vi "hts_commands.vi"(8 "Error IN":errorcluster, 9 "EXP SETTINGS":refnum<notifier>, 10 "SETTINGS":refnum<notifier>, 11 "COMMAND":T1) -> (0 "error out":errorcluster, 1 "EXP Settings":refnum<notifier>, 2 "Settings":refnum<notifier>)   [LabVIEW 2013]
uses:
  main_machine/type_defs/global_settings.ctl
  main_machine/type_defs/experiment_settings.ctl
  main_machine/type_defs/experiment_states.ctl
  type_defs/hts_command_list.ctl
panel:
  out "current command":T1
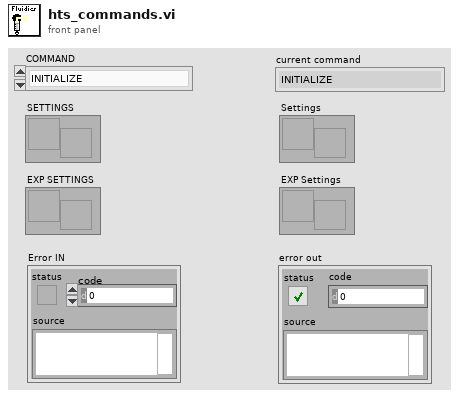
[diagram p1: front panel]
types:
  T1 = typedef "hts_command_list.ctl" = enum16{"INITIALIZE", "ADD MEDIA", "ADD INDUCER", "REMOVE CULTURE", "SAMPLE REACTOR", "CLEAR LINE TO VALVE", "CLEAR LINE TO CYTOMETER", "SAMPLE REACTOR NO DILUTION"}
  T2 = typedef "global_settings.ctl" = cluster{"# REACTORS":u32, "17X PORT":i32, "WASTE POSITION ":i32, "SECONDS BETWEEN SAMPLING":dbl, "FACS DIVA DIRECTORY":path, "DATA FILE":path, "REACTORS TO USE":u32[], "PULSE PERIOD":i32, "USE LIGHTS?":bool, "LED FILE":path, "LED CHANNELS":u32[], "PULSE LENGTH":i32, "SUMMARY FILE":path, "OUTGROWTH TIME POINTS":dbl, "SELECTION VALVE PORT":refnum<visa-resource-name>, "HTS PORT":refnum<visa-resource-name>, "DILUTION VOLUME (uL)":i32, "DILUTION FILE":path, "1X PORT":i32}
  T3 = typedef "experiment_settings.ctl" = cluster{"fcs file byte offset":i64, "LED Device Handle Out":u32, "START TIME":timestamp, "CURRENT VALVE":u32, "SAMPLE #":i32, "FCS FILE PATH":path, "TIME POINT":i32, "STATE":T4, "TIME TILL SAMPLE":dbl, "DILUTION  TABLE":dbl[][]}
  T4 = typedef "experiment_states.ctl" = enum16{"OUTGROWTH", "INDUCTION", "EXPERIMENT"}
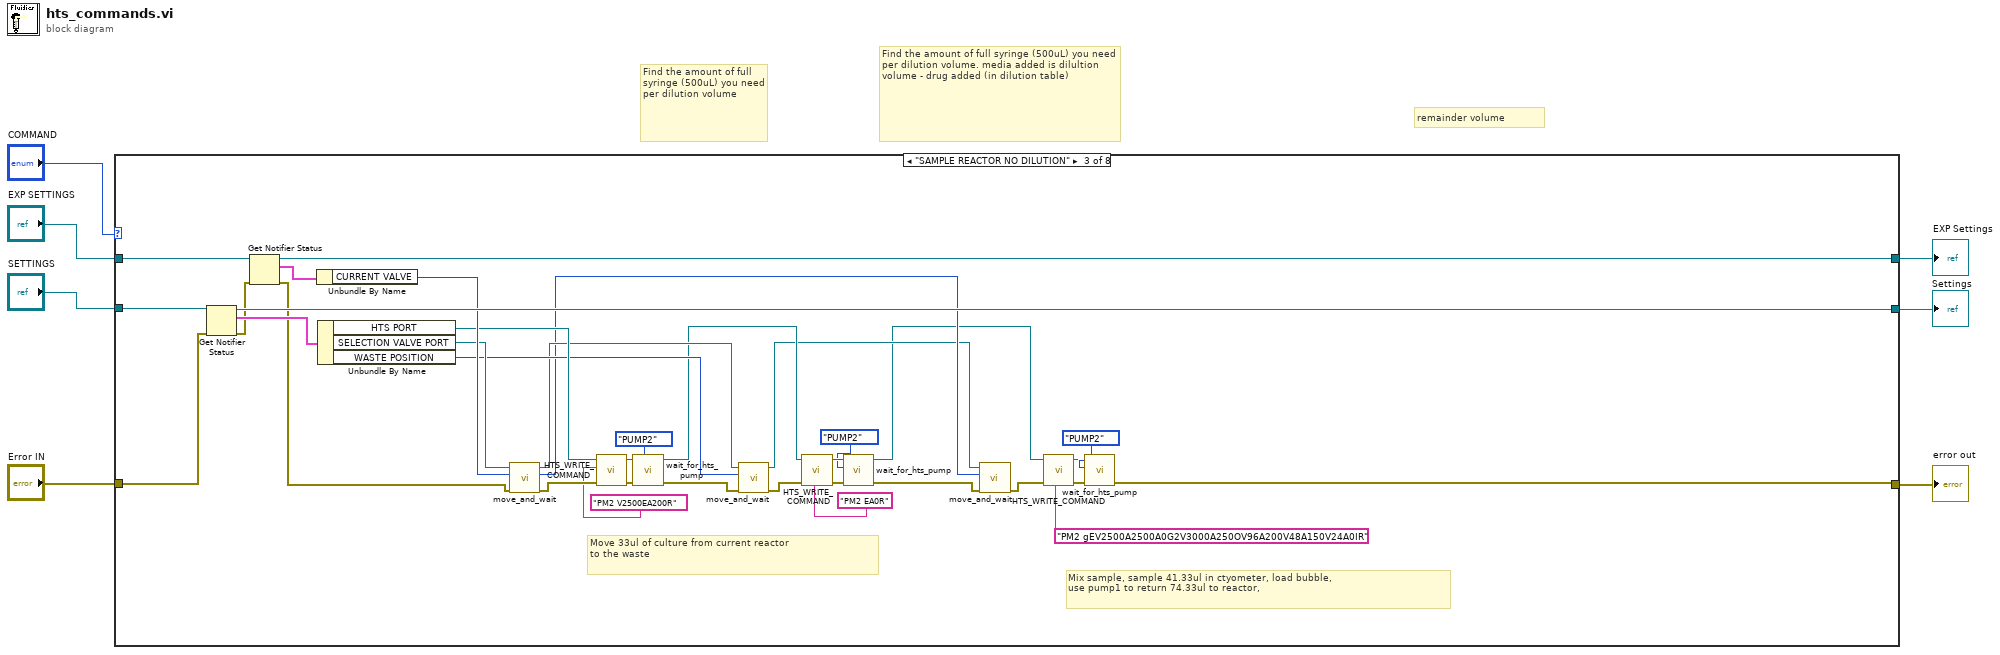
[diagram p0: block diagram]
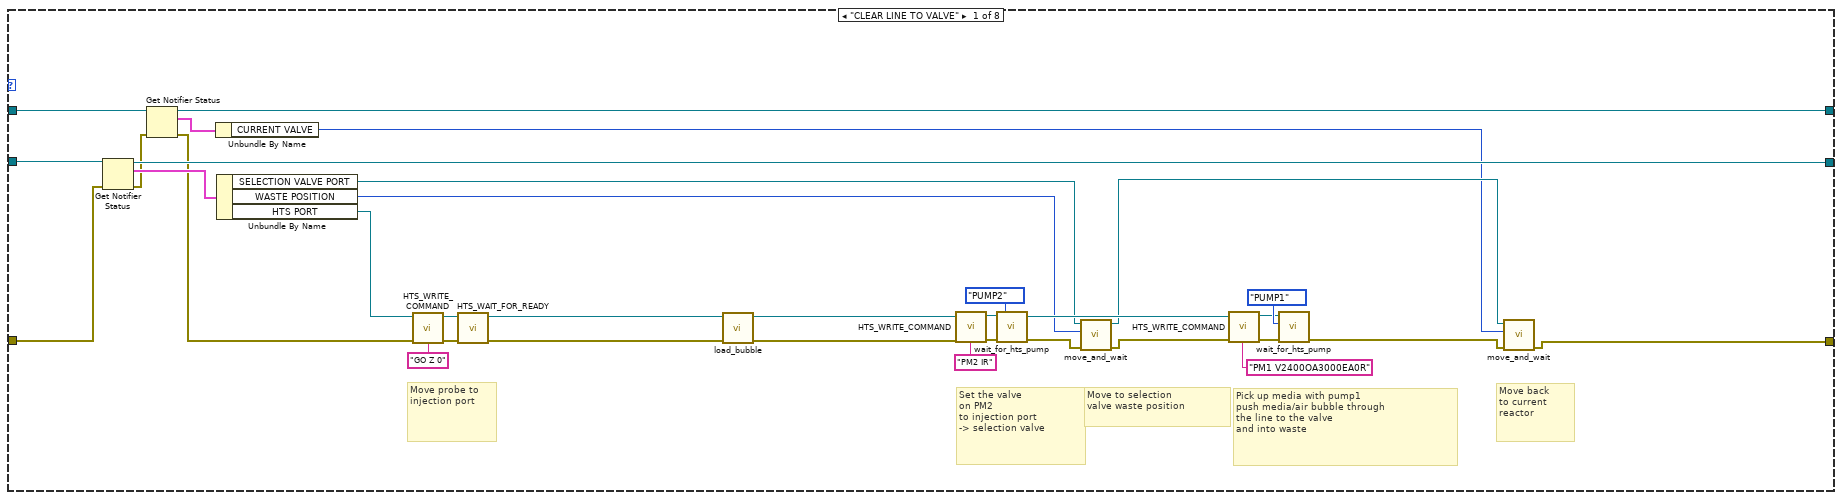
[diagram p2: hidden frame]
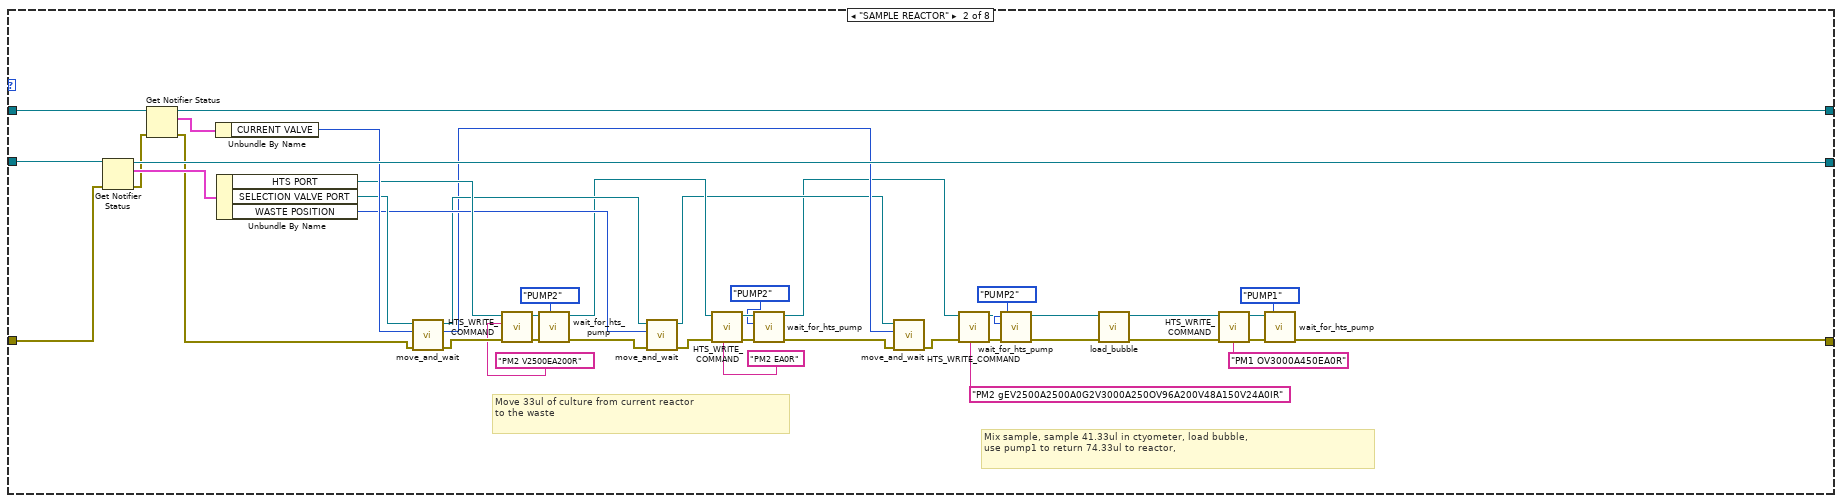
[diagram p3: hidden frame]
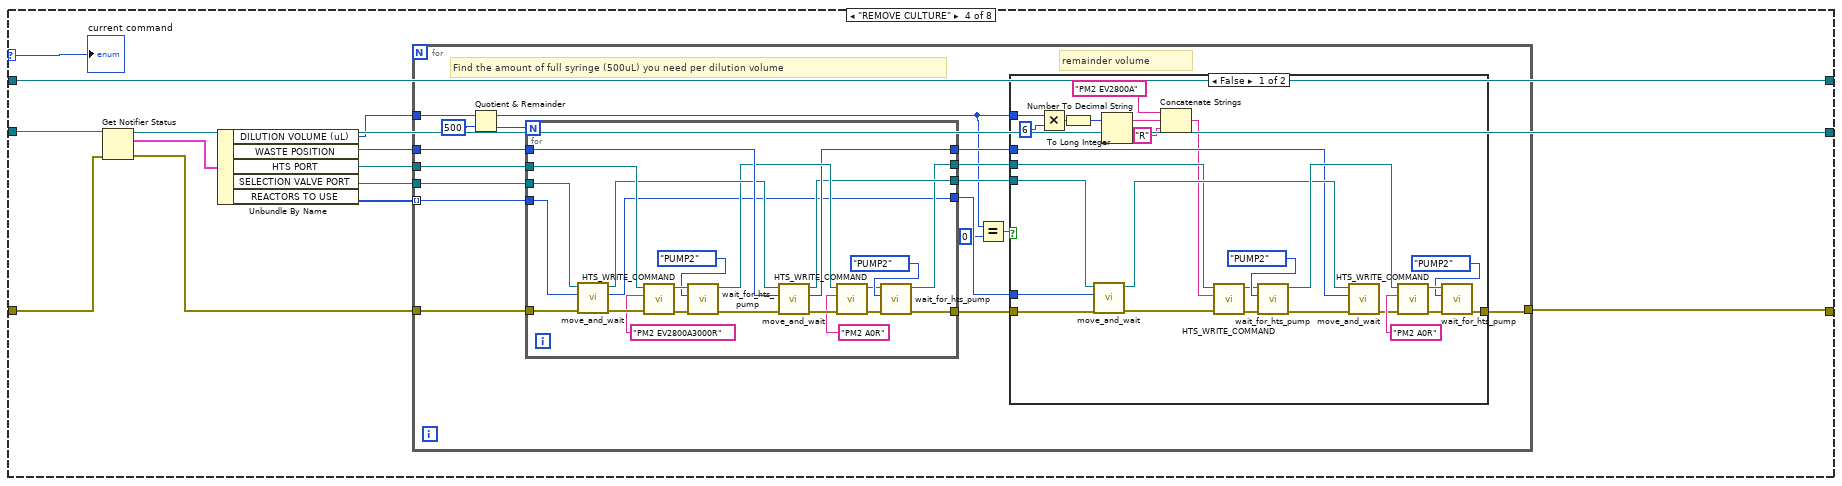
[diagram p4: hidden frame]
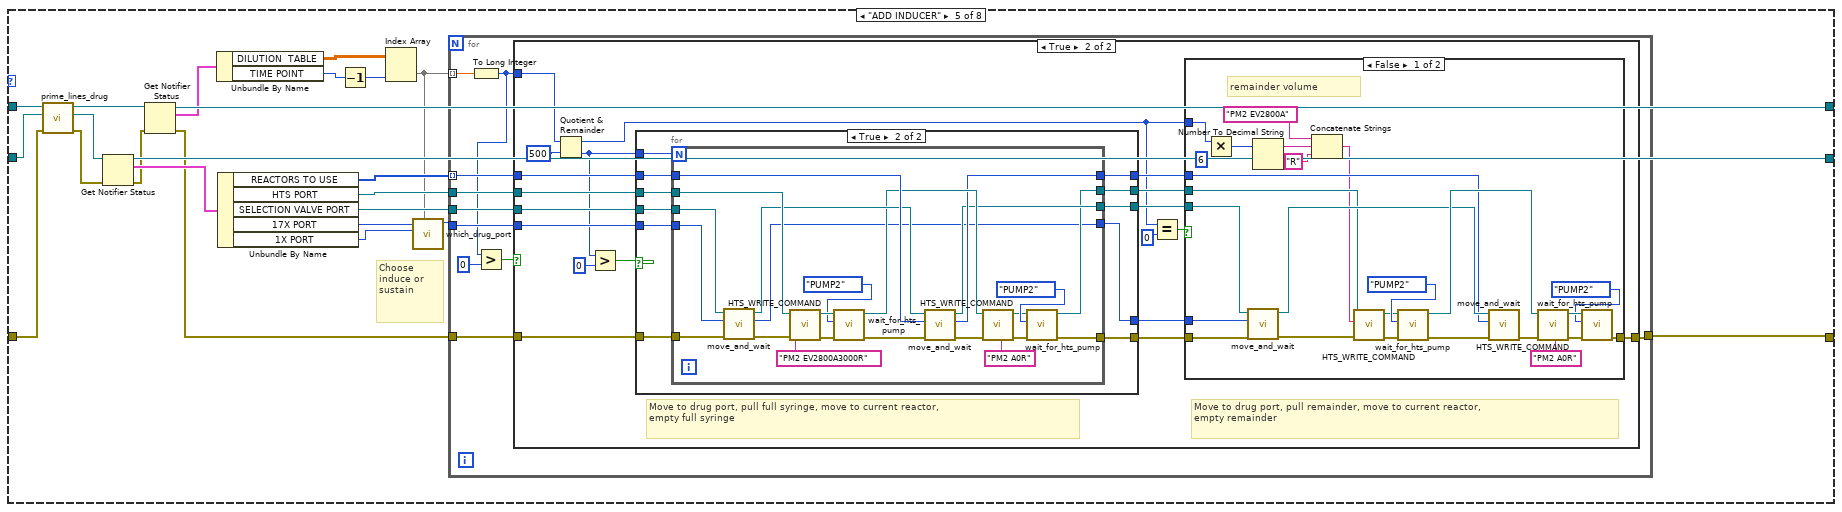
[diagram p6: hidden frame]
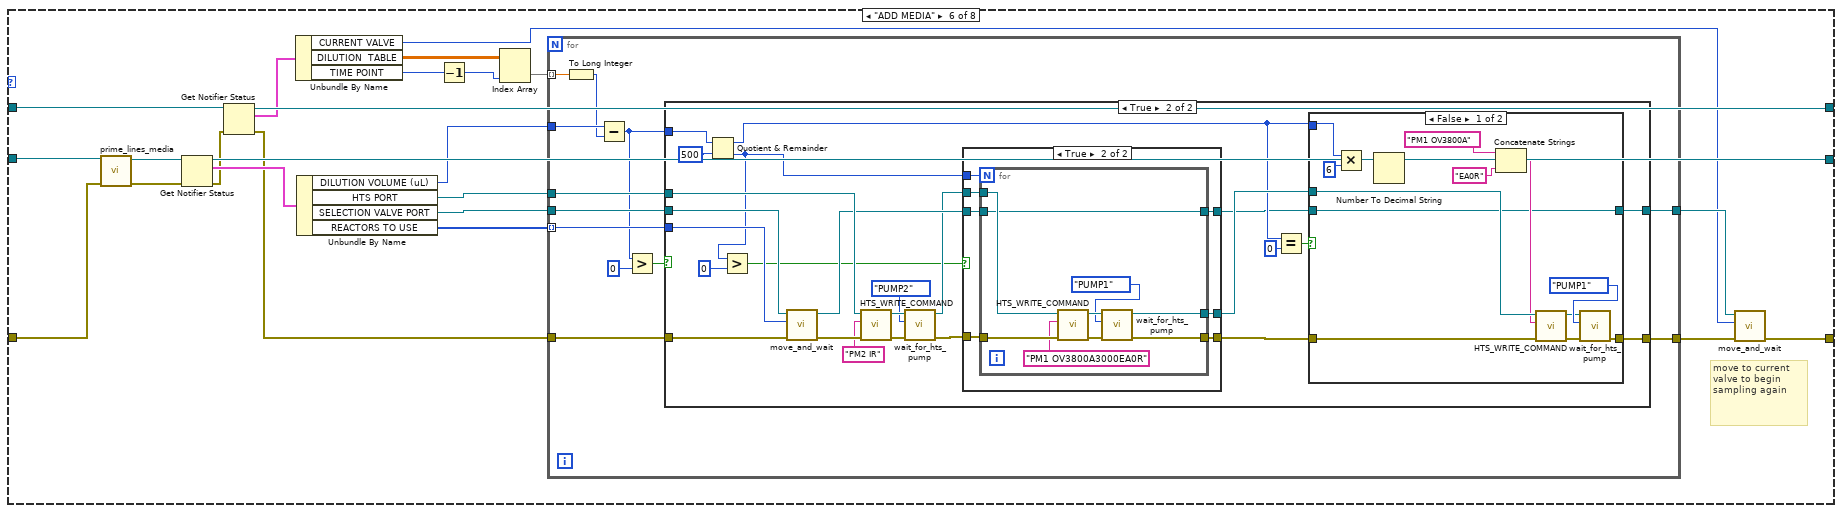
[diagram p10: hidden frame]
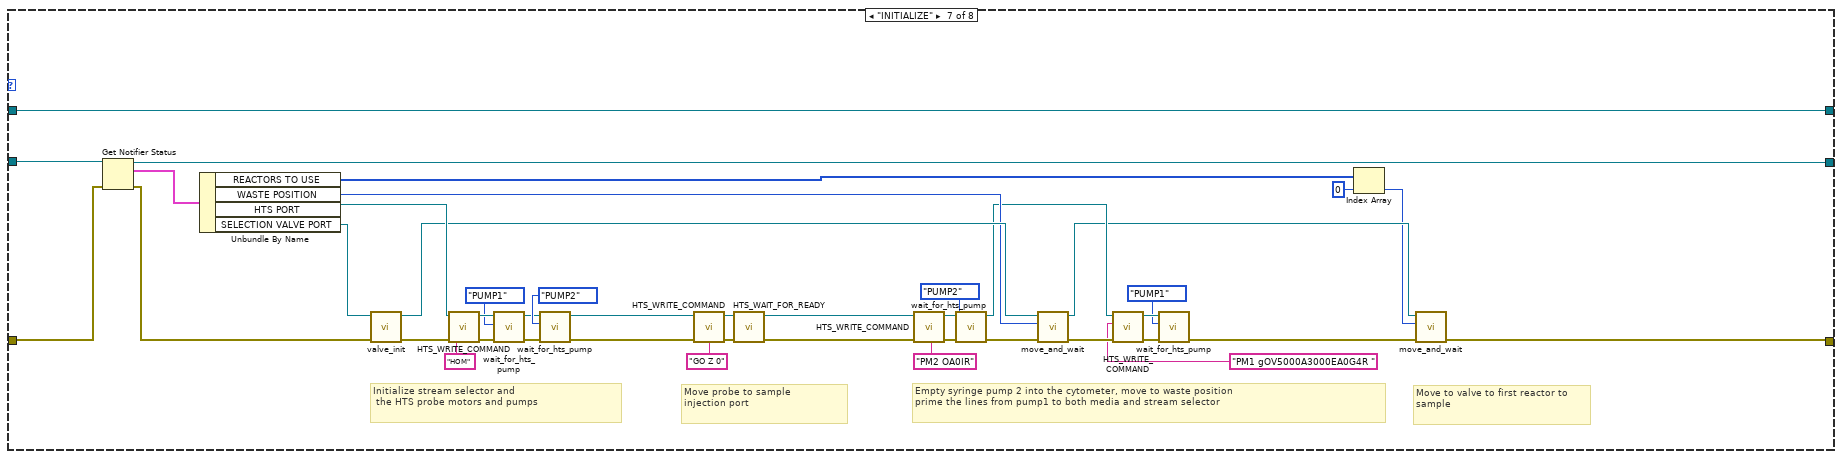
[diagram p14: hidden frame]
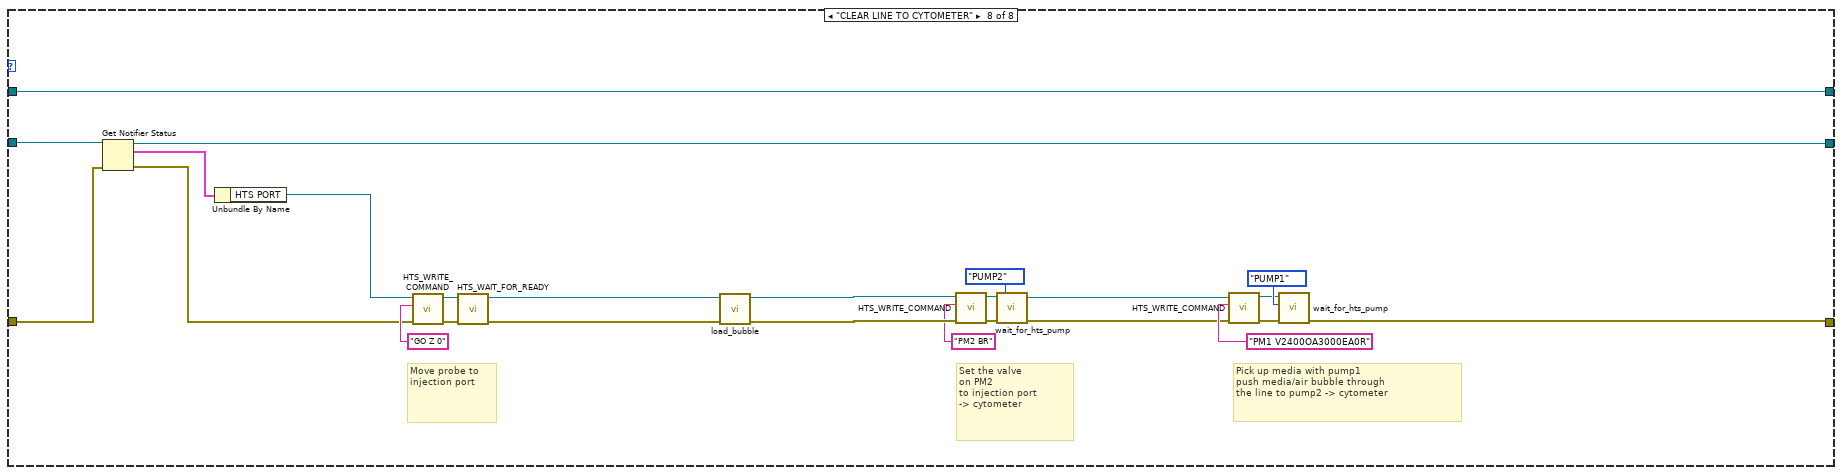
[diagram p15: hidden frame]
diagram:
  # "Find the amount of full syringe (500uL) you need per dilution volume"
  # "remainder volume"
  # "Find the amount of full syringe (500uL) you need per dilution volume. media added is dilultion volume - drug added (in dilution table)"
  n1 = case shown="\"SAMPLE REACTOR NO DILUTION\"" "COMMAND" {
    selector: "COMMAND" -> [_ _ _ w123 _ _ _ _]
    tunnel: [w26 w46 w86 w127 w220 w324 w418 w461] -> w6
    tunnel: "Error IN" -> [w24 w81 w117 w133 w208 w327 w457 w466]
    tunnel: "SETTINGS" -> [w25 w82 w118 w134 w211 w329 w458 w467]
    tunnel: "EXP SETTINGS" -> [w15 w77 w113 w126 w212 w339 w425 w460]
    tunnel: [w20 w79 w115 w124 w219 w340 w455 w464] -> w5
    tunnel: [w12 w75 w111 w126 w218 w338 w425 w460] -> w4
    frame "CLEAR LINE TO VALVE" {
      # "Move back\nto current \nreactor"
      # "Pick up media with pump1\npush media/air bubble through\nthe line to the valve \nand into waste"
      # "Move to selection \nvalve waste position"
      # "Set the valve \non PM2 \nto injection port\n-> selection valve"
      # "Move probe to injection port"
      n2 = Get Notifier Status(notifier=w25, error in (no error)=w24) -> (notifier out=w20:refnum<notifier>, current notification=w23:T2, error out=w17:errorcluster)  [unwired: 2 out]
      n3 = Get Notifier Status(notifier=w15, error in (no error)=w17) -> (notifier out=w12:refnum<notifier>, current notification=w14:T3, error out=w16:errorcluster)  [unwired: 2 out]
      n4 = Unbundle By Name(w14) -> ("CURRENT VALVE"=w13:u32)
      n5 = Unbundle By Name(w23) -> ("SELECTION VALVE PORT"=w22:refnum<visa-resource-name>, "WASTE POSITION"=w19:i32, "HTS PORT"=w18:refnum<visa-resource-name>)
      n6 = call "HTS_WRITE_COMMAND.vi"("Error IN"=w16, "Command"="GO Z 0", "HTS PORT IN"=w18) -> ("Error OUT"=w40:errorcluster, "HTS PORT OUT"=w41:refnum<visa-resource-name>)  [unwired: 6 in, 1 out]
      n7 = call "HTS_WAIT_FOR_READY.vi"("Error IN"=w40, "VISA resource IN"=w41) -> ("Error OUT"=w9:errorcluster, "VISA resource OUT"=w11:refnum<visa-resource-name>)  [unwired: 6 in, 2 out]
      n8 = call "load_bubble.vi"("error in (no error)"=w9, "HTS PORT"=w11) -> ("error out"=w8:errorcluster, "HTS PORT OUT"=w10:refnum<visa-resource-name>)  [unwired: 8 in]
      n9 = call "HTS_WRITE_COMMAND.vi"("Error IN"=w8, "Command"="PM2 IR", "HTS PORT IN"=w10) -> ("Error OUT"=w33:errorcluster, "HTS PORT OUT"=w34:refnum<visa-resource-name>)  [unwired: 6 in, 1 out]
      n10 = call "wait_for_hts_pump.vi"("error in (no error)"=w33, "PUMP"=enum16{"PUMP2", "PUMP1"}."PUMP2", "HTS PORT IN"=w34) -> ("error out"=w30:errorcluster, "HTS PORT OUT"=w29:refnum<visa-resource-name>)  [unwired: 7 in]
      n11 = call "move_and_wait.vi"("Error IN"=w30, "MOVE TO POSITION"=w19, "VISA Resource IN"=w22) -> ("Error OUT"=w28:errorcluster, "Visa Resource OUT"=w21:refnum<visa-resource-name>)  [unwired: 6 in, 1 out]
      n12 = call "HTS_WRITE_COMMAND.vi"("Error IN"=w28, "Command"="PM1 V2400OA3000EA0R", "HTS PORT IN"=w29) -> ("Error OUT"=w37:errorcluster, "HTS PORT OUT"=w36:refnum<visa-resource-name>)  [unwired: 6 in, 1 out]
      n13 = call "wait_for_hts_pump.vi"("error in (no error)"=w37, "PUMP"=enum16{"PUMP2", "PUMP1"}."PUMP1", "HTS PORT IN"=w36) -> ("error out"=w27:errorcluster)  [unwired: 7 in, 1 out]
      n14 = call "move_and_wait.vi"("Error IN"=w27, "MOVE TO POSITION"=w13, "VISA Resource IN"=w21) -> ("Error OUT"=w26:errorcluster)  [unwired: 6 in, 2 out]
    }
    frame "SAMPLE REACTOR" {
      # "Mix sample, sample 41.33ul in ctyometer, load bubble,\nuse pump1 to return 74.33ul to reactor,"
      # "Move 33ul of culture from current reactor\nto the waste"
      n15 = Get Notifier Status(notifier=w82, error in (no error)=w81) -> (notifier out=w79:refnum<notifier>, current notification=w80:T2, error out=w78:errorcluster)  [unwired: 2 out]
      n16 = Get Notifier Status(notifier=w77, error in (no error)=w78) -> (notifier out=w75:refnum<notifier>, current notification=w76:T3, error out=w73:errorcluster)  [unwired: 2 out]
      n17 = Unbundle By Name(w76) -> ("CURRENT VALVE"=w74:u32)
      n18 = Unbundle By Name(w80) -> ("HTS PORT"=w71:refnum<visa-resource-name>, "SELECTION VALVE PORT"=w70:refnum<visa-resource-name>, "WASTE POSITION"=w63:i32)
      n19 = call "move_and_wait.vi"("Error IN"=w73, "MOVE TO POSITION"=w74, "VISA Resource IN"=w70) -> ("Error OUT"=w72:errorcluster, "CURRENT POSITION"=w55:i32, "Visa Resource OUT"=w62:refnum<visa-resource-name>)  [unwired: 6 in]
      n20 = call "HTS_WRITE_COMMAND.vi"("Error IN"=w72, "Command"="PM2 V2500EA200R", "HTS PORT IN"=w71) -> ("Error OUT"=w84:errorcluster, "HTS PORT OUT"=w85:refnum<visa-resource-name>)  [unwired: 6 in, 1 out]
      n21 = call "wait_for_hts_pump.vi"("error in (no error)"=w84, "PUMP"=enum16{"PUMP2", "PUMP1"}."PUMP2", "HTS PORT IN"=w85) -> ("error out"=w64:errorcluster, "HTS PORT OUT"=w60:refnum<visa-resource-name>)  [unwired: 7 in]
      n22 = call "move_and_wait.vi"("Error IN"=w64, "MOVE TO POSITION"=w63, "VISA Resource IN"=w62) -> ("Error OUT"=w61:errorcluster, "Visa Resource OUT"=w54:refnum<visa-resource-name>)  [unwired: 6 in, 1 out]
      n23 = call "HTS_WRITE_COMMAND.vi"("Error IN"=w61, "Command"="PM2 EA0R", "HTS PORT IN"=w60) -> ("Error OUT"=w68:errorcluster, "HTS PORT OUT"=w67:refnum<visa-resource-name>)  [unwired: 6 in, 1 out]
      n24 = call "wait_for_hts_pump.vi"("error in (no error)"=w68, "PUMP"=enum16{"PUMP2", "PUMP1"}."PUMP2", "HTS PORT IN"=w67) -> ("error out"=w53:errorcluster, "HTS PORT OUT"=w51:refnum<visa-resource-name>)  [unwired: 7 in]
      n25 = call "move_and_wait.vi"("Error IN"=w53, "MOVE TO POSITION"=w55, "VISA Resource IN"=w54) -> ("Error OUT"=w52:errorcluster)  [unwired: 6 in, 2 out]
      n26 = call "HTS_WRITE_COMMAND.vi"("Error IN"=w52, "Command"="PM2 gEV2500A2500A0G2V3000A250OV96A200V48A150V24A0IR", "HTS PORT IN"=w51) -> ("Error OUT"=w56:errorcluster, "HTS PORT OUT"=w57:refnum<visa-resource-name>)  [unwired: 6 in, 1 out]
      n27 = call "wait_for_hts_pump.vi"("error in (no error)"=w56, "PUMP"=enum16{"PUMP2", "PUMP1"}."PUMP2", "HTS PORT IN"=w57) -> ("error out"=w43:errorcluster, "HTS PORT OUT"=w45:refnum<visa-resource-name>)  [unwired: 7 in]
      n28 = call "load_bubble.vi"("error in (no error)"=w43, "HTS PORT"=w45) -> ("error out"=w42:errorcluster, "HTS PORT OUT"=w44:refnum<visa-resource-name>)  [unwired: 8 in]
      n29 = call "HTS_WRITE_COMMAND.vi"("Error IN"=w42, "Command"="PM1 OV3000A450EA0R", "HTS PORT IN"=w44) -> ("Error OUT"=w50:errorcluster, "HTS PORT OUT"=w49:refnum<visa-resource-name>)  [unwired: 6 in, 1 out]
      n30 = call "wait_for_hts_pump.vi"("error in (no error)"=w50, "PUMP"=enum16{"PUMP2", "PUMP1"}."PUMP1", "HTS PORT IN"=w49) -> ("error out"=w46:errorcluster)  [unwired: 7 in, 1 out]
    }
    frame "SAMPLE REACTOR NO DILUTION" {
      # "Mix sample, sample 41.33ul in ctyometer, load bubble,\nuse pump1 to return 74.33ul to reactor,"
      # "Move 33ul of culture from current reactor\nto the waste"
      n31 = Get Notifier Status(notifier=w118, error in (no error)=w117) -> (notifier out=w115:refnum<notifier>, current notification=w116:T2, error out=w114:errorcluster)  [unwired: 2 out]
      n32 = Get Notifier Status(notifier=w113, error in (no error)=w114) -> (notifier out=w111:refnum<notifier>, current notification=w112:T3, error out=w109:errorcluster)  [unwired: 2 out]
      n33 = Unbundle By Name(w112) -> ("CURRENT VALVE"=w110:u32)
      n34 = Unbundle By Name(w116) -> ("HTS PORT"=w107:refnum<visa-resource-name>, "SELECTION VALVE PORT"=w106:refnum<visa-resource-name>, "WASTE POSITION"=w99:i32)
      n35 = call "move_and_wait.vi"("Error IN"=w109, "MOVE TO POSITION"=w110, "VISA Resource IN"=w106) -> ("Error OUT"=w108:errorcluster, "CURRENT POSITION"=w91:i32, "Visa Resource OUT"=w98:refnum<visa-resource-name>)  [unwired: 6 in]
      n36 = call "HTS_WRITE_COMMAND.vi"("Error IN"=w108, "Command"="PM2 V2500EA200R", "HTS PORT IN"=w107) -> ("Error OUT"=w120:errorcluster, "HTS PORT OUT"=w121:refnum<visa-resource-name>)  [unwired: 6 in, 1 out]
      n37 = call "wait_for_hts_pump.vi"("error in (no error)"=w120, "PUMP"=enum16{"PUMP2", "PUMP1"}."PUMP2", "HTS PORT IN"=w121) -> ("error out"=w100:errorcluster, "HTS PORT OUT"=w96:refnum<visa-resource-name>)  [unwired: 7 in]
      n38 = call "move_and_wait.vi"("Error IN"=w100, "MOVE TO POSITION"=w99, "VISA Resource IN"=w98) -> ("Error OUT"=w97:errorcluster, "Visa Resource OUT"=w90:refnum<visa-resource-name>)  [unwired: 6 in, 1 out]
      n39 = call "HTS_WRITE_COMMAND.vi"("Error IN"=w97, "Command"="PM2 EA0R", "HTS PORT IN"=w96) -> ("Error OUT"=w104:errorcluster, "HTS PORT OUT"=w103:refnum<visa-resource-name>)  [unwired: 6 in, 1 out]
      n40 = call "wait_for_hts_pump.vi"("error in (no error)"=w104, "PUMP"=enum16{"PUMP2", "PUMP1"}."PUMP2", "HTS PORT IN"=w103) -> ("error out"=w89:errorcluster, "HTS PORT OUT"=w87:refnum<visa-resource-name>)  [unwired: 7 in]
      n41 = call "move_and_wait.vi"("Error IN"=w89, "MOVE TO POSITION"=w91, "VISA Resource IN"=w90) -> ("Error OUT"=w88:errorcluster)  [unwired: 6 in, 2 out]
      n42 = call "HTS_WRITE_COMMAND.vi"("Error IN"=w88, "Command"="PM2 gEV2500A2500A0G2V3000A250OV96A200V48A150V24A0IR", "HTS PORT IN"=w87) -> ("Error OUT"=w92:errorcluster, "HTS PORT OUT"=w93:refnum<visa-resource-name>)  [unwired: 6 in, 1 out]
      n43 = call "wait_for_hts_pump.vi"("error in (no error)"=w92, "PUMP"=enum16{"PUMP2", "PUMP1"}."PUMP2", "HTS PORT IN"=w93) -> ("error out"=w86:errorcluster)  [unwired: 7 in, 1 out]
    }
    frame "REMOVE CULTURE" {
      n44 = Get Notifier Status(notifier=w134, error in (no error)=w133) -> (notifier out=w124:refnum<notifier>, current notification=w132:T2, error out=w125:errorcluster)  [unwired: 2 out]
      n45 = Unbundle By Name(w132) -> ("DILUTION VOLUME (uL)"=w122:i32, "WASTE POSITION"=w128:i32, "HTS PORT"=w129:refnum<visa-resource-name>, "SELECTION VALVE PORT"=w130:refnum<visa-resource-name>, "REACTORS TO USE"=w131:u32[])
      n46 = for {
        tunnel: w125 -> [w151]
        tunnel: w131 -> [w150] mode=indexing
        tunnel: w130 -> [w149]
        tunnel: w129 -> [w148]
        tunnel: w128 -> [w147]
        tunnel: w122 -> [w146]
        tunnel: [w138] -> w127
        # "remainder volume"
        # "Find the amount of full syringe (500uL) you need per dilution volume"
        n47 = Quotient & Remainder(x=w146, y=500) -> (x-y*floor(x/y)=w136:i32, floor(x/y)=w144:i32)
        n48 = for {
          N: w144 -> [_]
          tunnel: w151 -> [w201]
          tunnel: w150 -> [w200]
          tunnel: w149 -> [w199]
          tunnel: w148 -> [w197]
          tunnel: w147 -> [w189]
          tunnel: [w183] -> w143
          tunnel: [w182] -> w141
          tunnel: [w181] -> w142
          tunnel: [w180] -> w139
          tunnel: [w179] -> w140
          n49 = call "move_and_wait.vi"("Error IN"=w201, "MOVE TO POSITION"=w200, "VISA Resource IN"=w199) -> ("Error OUT"=w198:errorcluster, "CURRENT POSITION"=w179:i32, "Visa Resource OUT"=w188:refnum<visa-resource-name>)  [unwired: 6 in]
          n50 = call "HTS_WRITE_COMMAND.vi"("Error IN"=w198, "Command"="PM2 EV2800A3000R", "HTS PORT IN"=w197) -> ("Error OUT"=w195:errorcluster, "HTS PORT OUT"=w196:refnum<visa-resource-name>)  [unwired: 6 in, 1 out]
          n51 = call "wait_for_hts_pump.vi"("error in (no error)"=w195, "PUMP"=enum16{"PUMP2", "PUMP1"}."PUMP2", "HTS PORT IN"=w196) -> ("error out"=w190:errorcluster, "HTS PORT OUT"=w187:refnum<visa-resource-name>)  [unwired: 7 in]
          n52 = call "move_and_wait.vi"("Error IN"=w190, "MOVE TO POSITION"=w189, "VISA Resource IN"=w188) -> ("Error OUT"=w186:errorcluster, "CURRENT POSITION"=w183:i32, "Visa Resource OUT"=w182:refnum<visa-resource-name>)  [unwired: 6 in]
          n53 = call "HTS_WRITE_COMMAND.vi"("Error IN"=w186, "Command"="PM2 A0R", "HTS PORT IN"=w187) -> ("Error OUT"=w192:errorcluster, "HTS PORT OUT"=w191:refnum<visa-resource-name>)  [unwired: 6 in, 1 out]
          n54 = call "wait_for_hts_pump.vi"("error in (no error)"=w192, "PUMP"=enum16{"PUMP2", "PUMP1"}."PUMP2", "HTS PORT IN"=w191) -> ("error out"=w180:errorcluster, "HTS PORT OUT"=w181:refnum<visa-resource-name>)  [unwired: 7 in]
        }
        n55 = Equal?(x=w136, y=0) -> (x = y?=w137:bool)
        n56 = case shown="False" w137 {
          tunnel: w143 -> [w165 _]
          tunnel: w142 -> [w164 _]
          tunnel: w141 -> [w163 _]
          tunnel: w140 -> [w162 _]
          tunnel: w139 -> [w161 w178]
          tunnel: w136 -> [w160 _]
          tunnel: [w152 w178] -> w138
          frame False {
            n57 = Multiply(x=w160, y=6) -> (x*y=w156:i32)
            n58 = To Long Integer(number=w156) -> (32bit integer=w155:i32)
            n59 = call "move_and_wait.vi"("Error IN"=w161, "MOVE TO POSITION"=w162, "VISA Resource IN"=w163) -> ("Error OUT"=w166:errorcluster, "Visa Resource OUT"=w174:refnum<visa-resource-name>)  [unwired: 6 in, 1 out]
            n60 = Number To Decimal String(number=w155) -> (decimal integer string=w158:string)  [unwired: 1 in]
            n61 = Concatenate Strings("PM2 EV2800A" ("Command"), w158, "R" ("string")) -> (w153:string)
            n62 = call "HTS_WRITE_COMMAND.vi"("Error IN"=w166, "Command"=w153, "HTS PORT IN"=w164) -> ("Error OUT"=w168:errorcluster, "HTS PORT OUT"=w167:refnum<visa-resource-name>)  [unwired: 6 in, 1 out]
            n63 = call "wait_for_hts_pump.vi"("error in (no error)"=w168, "PUMP"=enum16{"PUMP2", "PUMP1"}."PUMP2", "HTS PORT IN"=w167) -> ("error out"=w173:errorcluster, "HTS PORT OUT"=w175:refnum<visa-resource-name>)  [unwired: 7 in]
            n64 = call "move_and_wait.vi"("Error IN"=w173, "MOVE TO POSITION"=w165, "VISA Resource IN"=w174) -> ("Error OUT"=w176:errorcluster)  [unwired: 6 in, 2 out]
            n65 = call "HTS_WRITE_COMMAND.vi"("Error IN"=w176, "Command"="PM2 A0R", "HTS PORT IN"=w175) -> ("Error OUT"=w171:errorcluster, "HTS PORT OUT"=w172:refnum<visa-resource-name>)  [unwired: 6 in, 1 out]
            n66 = call "wait_for_hts_pump.vi"("error in (no error)"=w171, "PUMP"=enum16{"PUMP2", "PUMP1"}."PUMP2", "HTS PORT IN"=w172) -> ("error out"=w152:errorcluster)  [unwired: 7 in, 1 out]
          }
          frame True {
          }
        }
      }
      "current command" <- w123
    }
    frame "ADD INDUCER" {
      # "Choose induce or sustain"
      n67 = call "prime_lines_drug.vi"("error in (no error)"=w208, "GLOBAL SETTINGS IN"=w211, "EXP SETTINGS IN"=w212) -> ("error out"=w207:errorcluster, "GLOBAL SETTINGS OUT"=w210:refnum<notifier>, "EXP SETTINGS OUT"=w209:refnum<notifier>)  [unwired: 6 in]
      n68 = Get Notifier Status(notifier=w210, error in (no error)=w207) -> (notifier out=w219:refnum<notifier>, current notification=w224:T2, error out=w217:errorcluster)  [unwired: 2 out]
      n69 = Get Notifier Status(notifier=w209, error in (no error)=w217) -> (notifier out=w218:refnum<notifier>, current notification=w215:T3, error out=w216:errorcluster)  [unwired: 2 out]
      n70 = Unbundle By Name(w215) -> ("DILUTION  TABLE"=w214:dbl[][], "TIME POINT"=w213:i32)
      n71 = Unbundle By Name(w224) -> ("REACTORS TO USE"=w221:u32[], "HTS PORT"=w222:refnum<visa-resource-name>, "SELECTION VALVE PORT"=w223:refnum<visa-resource-name>, "17X PORT"=w205:i32, "1X PORT"=w204:i32)
      n72 = Decrement(x=w213) -> (x-1=w206:i32)
      n73 = Index Array(array=w214, index (col)=w206) -> (element=w202:dbl[])  [unwired: 1 in]
      n74 = call "which_drug_port.vi"("DILUTION COLUMN"=w202, "1X PORT"=w204, "17X PORT"=w205) -> ("DRUG PORT"=w203:i32)  [unwired: 8 in]
      n75 = for {
        tunnel: w216 -> [w234]
        tunnel: w223 -> [w233]
        tunnel: w222 -> [w232]
        tunnel: w221 -> [w231] mode=indexing
        tunnel: [w230] -> w220
        tunnel: w202 -> [w229] mode=indexing
        tunnel: w203 -> [w228]
        n76 = To Long Integer(number=w229) -> (32bit integer=w226:i32)
        n77 = Greater?(x=w226, y=0) -> (0:w227:bool)
        n78 = case shown="True" w227 {
          tunnel: w234 -> [w235 w254]
          tunnel: w233 -> [_ w253]
          tunnel: w232 -> [_ w252]
          tunnel: w231 -> [_ w251]
          tunnel: [w235 w244] -> w230
          tunnel: w228 -> [_ w243]
          tunnel: w226 -> [_ w242]
          frame False {
          }
          frame True {
            # "Move to drug port, pull remainder, move to current reactor,\nempty remainder"
            # "Move to drug port, pull full syringe, move to current reactor,\nempty full syringe"
            n79 = Quotient & Remainder(x=w242, y=500) -> (x-y*floor(x/y)=w237:i32, floor(x/y)=w239:i32)
            n80 = Greater?(x=w239, y=0) -> (0:w240:bool)
            n81 = case shown="True" w240 {
              tunnel: w254 -> [w282 w296]
              tunnel: w253 -> [w285 w295]
              tunnel: w252 -> [w284 w294]
              tunnel: w251 -> [w283 w293]
              tunnel: w239 -> [_ w292]
              tunnel: [w283 w291] -> w249
              tunnel: [w284 w290] -> w248
              tunnel: [w285 w289] -> w247
              tunnel: [w281 w288] -> w246
              tunnel: [w282 w287] -> w245
              tunnel: w243 -> [w281 w286]
              frame False {
              }
              frame True {
                n82 = for {
                  N: w292 -> [_]
                  tunnel: w296 -> [w319]
                  tunnel: w295 -> [w318]
                  tunnel: w294 -> [w316]
                  tunnel: w293 -> [w308]
                  tunnel: [w302] -> w291
                  tunnel: [w301] -> w289
                  tunnel: [w300] -> w290
                  tunnel: [w299] -> w287
                  tunnel: [w298] -> w288
                  tunnel: w286 -> [w297]
                  n83 = call "move_and_wait.vi"("Error IN"=w319, "MOVE TO POSITION"=w297, "VISA Resource IN"=w318) -> ("Error OUT"=w317:errorcluster, "CURRENT POSITION"=w298:i32, "Visa Resource OUT"=w307:refnum<visa-resource-name>)  [unwired: 6 in]
                  n84 = call "HTS_WRITE_COMMAND.vi"("Error IN"=w317, "Command"="PM2 EV2800A3000R", "HTS PORT IN"=w316) -> ("Error OUT"=w314:errorcluster, "HTS PORT OUT"=w315:refnum<visa-resource-name>)  [unwired: 6 in, 1 out]
                  n85 = call "wait_for_hts_pump.vi"("error in (no error)"=w314, "PUMP"=enum16{"PUMP2", "PUMP1"}."PUMP2", "HTS PORT IN"=w315) -> ("error out"=w309:errorcluster, "HTS PORT OUT"=w306:refnum<visa-resource-name>)  [unwired: 7 in]
                  n86 = call "move_and_wait.vi"("Error IN"=w309, "MOVE TO POSITION"=w308, "VISA Resource IN"=w307) -> ("Error OUT"=w305:errorcluster, "CURRENT POSITION"=w302:i32, "Visa Resource OUT"=w301:refnum<visa-resource-name>)  [unwired: 6 in]
                  n87 = call "HTS_WRITE_COMMAND.vi"("Error IN"=w305, "Command"="PM2 A0R", "HTS PORT IN"=w306) -> ("Error OUT"=w311:errorcluster, "HTS PORT OUT"=w310:refnum<visa-resource-name>)  [unwired: 6 in, 1 out]
                  n88 = call "wait_for_hts_pump.vi"("error in (no error)"=w311, "PUMP"=enum16{"PUMP2", "PUMP1"}."PUMP2", "HTS PORT IN"=w310) -> ("error out"=w299:errorcluster, "HTS PORT OUT"=w300:refnum<visa-resource-name>)  [unwired: 7 in]
                }
              }
            }
            n89 = Equal?(x=w237, y=0) -> (x = y?=w238:bool)
            n90 = case shown="False" w238 {
              tunnel: w249 -> [w267 _]
              tunnel: w248 -> [w266 _]
              tunnel: w247 -> [w265 _]
              tunnel: w246 -> [w264 _]
              tunnel: w245 -> [w263 w280]
              tunnel: [w258 w280] -> w244
              tunnel: w237 -> [w255 _]
              frame False {
                # "remainder volume"
                n91 = Multiply(x=w255, y=6) -> (x*y=w257:i32)
                n92 = call "move_and_wait.vi"("Error IN"=w263, "MOVE TO POSITION"=w264, "VISA Resource IN"=w265) -> ("Error OUT"=w268:errorcluster, "Visa Resource OUT"=w276:refnum<visa-resource-name>)  [unwired: 6 in, 1 out]
                n93 = Number To Decimal String(number=w257) -> (decimal integer string=w261:string)  [unwired: 1 in]
                n94 = Concatenate Strings("PM2 EV2800A" ("Command"), w261, "R" ("string")) -> (w259:string)
                n95 = call "HTS_WRITE_COMMAND.vi"("Error IN"=w268, "Command"=w259, "HTS PORT IN"=w266) -> ("Error OUT"=w270:errorcluster, "HTS PORT OUT"=w269:refnum<visa-resource-name>)  [unwired: 6 in, 1 out]
                n96 = call "wait_for_hts_pump.vi"("error in (no error)"=w270, "PUMP"=enum16{"PUMP2", "PUMP1"}."PUMP2", "HTS PORT IN"=w269) -> ("error out"=w275:errorcluster, "HTS PORT OUT"=w277:refnum<visa-resource-name>)  [unwired: 7 in]
                n97 = call "move_and_wait.vi"("Error IN"=w275, "MOVE TO POSITION"=w267, "VISA Resource IN"=w276) -> ("Error OUT"=w278:errorcluster)  [unwired: 6 in, 2 out]
                n98 = call "HTS_WRITE_COMMAND.vi"("Error IN"=w278, "Command"="PM2 A0R", "HTS PORT IN"=w277) -> ("Error OUT"=w273:errorcluster, "HTS PORT OUT"=w274:refnum<visa-resource-name>)  [unwired: 6 in, 1 out]
                n99 = call "wait_for_hts_pump.vi"("error in (no error)"=w273, "PUMP"=enum16{"PUMP2", "PUMP1"}."PUMP2", "HTS PORT IN"=w274) -> ("error out"=w258:errorcluster)  [unwired: 7 in, 1 out]
              }
              frame True {
              }
            }
          }
        }
      }
    }
    frame "ADD MEDIA" {
      # "move to current valve to begin sampling again"
      n100 = call "prime_lines_media.vi"("error in (no error)"=w327, "GLOBAL SETTINGS IN"=w329) -> ("error out"=w326:errorcluster, "GLOBAL SETTINGS OUT"=w328:refnum<notifier>)  [unwired: 8 in]
      n101 = Get Notifier Status(notifier=w328, error in (no error)=w326) -> (notifier out=w340:refnum<notifier>, current notification=w342:T2, error out=w337:errorcluster)  [unwired: 2 out]
      n102 = Get Notifier Status(notifier=w339, error in (no error)=w337) -> (notifier out=w338:refnum<notifier>, current notification=w336:T3, error out=w331:errorcluster)  [unwired: 2 out]
      n103 = Unbundle By Name(w336) -> ("CURRENT VALVE"=w322:u32, "DILUTION  TABLE"=w335:dbl[][], "TIME POINT"=w332:i32)
      n104 = Unbundle By Name(w342) -> ("DILUTION VOLUME (uL)"=w334:i32, "HTS PORT"=w330:refnum<visa-resource-name>, "SELECTION VALVE PORT"=w341:refnum<visa-resource-name>, "REACTORS TO USE"=w333:u32[])
      n105 = Decrement(x=w332) -> (x-1=w320:i32)
      n106 = Index Array(array=w335, index (col)=w320) -> (element=w321:dbl[])  [unwired: 1 in]
      n107 = for {
        tunnel: w331 -> [w354]
        tunnel: w341 -> [w353]
        tunnel: w330 -> [w352]
        tunnel: w321 -> [w351] mode=indexing
        tunnel: w334 -> [w350]
        tunnel: w333 -> [w348] mode=indexing
        tunnel: [w347] -> w325
        tunnel: [w346] -> w323
        n108 = To Long Integer(number=w351) -> (32bit integer=w349:i32)
        n109 = Subtract(x=w350, y=w349) -> (x-y=w343:i32)
        n110 = Greater?(x=w343, y=0) -> (0:w344:bool)
        n111 = case shown="True" w344 {
          tunnel: w354 -> [w355 w373]
          tunnel: w353 -> [w356 w381]
          tunnel: w352 -> [_ w380]
          tunnel: w348 -> [_ w377]
          tunnel: [w355 w375] -> w347
          tunnel: [w356 w366] -> w346
          tunnel: w343 -> [_ w374]
          frame False {
          }
          frame True {
            n112 = Quotient & Remainder(x=w374, y=500) -> (x-y*floor(x/y)=w369:i32, floor(x/y)=w372:i32)
            n113 = Greater?(x=w372, y=0) -> (0:w357:bool)
            n114 = call "move_and_wait.vi"("Error IN"=w373, "MOVE TO POSITION"=w377, "VISA Resource IN"=w381) -> ("Error OUT"=w360:errorcluster, "Visa Resource OUT"=w365:refnum<visa-resource-name>)  [unwired: 6 in, 1 out]
            n115 = call "HTS_WRITE_COMMAND.vi"("Error IN"=w360, "Command"="PM2 IR", "HTS PORT IN"=w380) -> ("Error OUT"=w364:errorcluster, "HTS PORT OUT"=w363:refnum<visa-resource-name>)  [unwired: 6 in, 1 out]
            n116 = call "wait_for_hts_pump.vi"("error in (no error)"=w364, "PUMP"=enum16{"PUMP2", "PUMP1"}."PUMP2", "HTS PORT IN"=w363) -> ("error out"=w361:errorcluster, "HTS PORT OUT"=w362:refnum<visa-resource-name>)  [unwired: 7 in]
            n117 = case shown="True" w357 {
              tunnel: [w382 w391] -> w378
              tunnel: [w384 w390] -> w376
              tunnel: w372 -> [_ w389]
              tunnel: [w383 w388] -> w367
              tunnel: w365 -> [w383 w387]
              tunnel: w362 -> [w382 w386]
              tunnel: w361 -> [w384 w385]
              frame False {
              }
              frame True {
                n118 = for {
                  N: w389 -> [_]
                  tunnel: w386 -> [w400]
                  tunnel: [w399] -> w391
                  tunnel: w385 -> [w397]
                  tunnel: [w398] -> w390
                  tunnel: w387 -> [w392]
                  tunnel: [w392] -> w388
                  n119 = call "HTS_WRITE_COMMAND.vi"("Error IN"=w397, "Command"="PM1 OV3800A3000EA0R", "HTS PORT IN"=w400) -> ("Error OUT"=w395:errorcluster, "HTS PORT OUT"=w396:refnum<visa-resource-name>)  [unwired: 6 in, 1 out]
                  n120 = call "wait_for_hts_pump.vi"("error in (no error)"=w395, "PUMP"=enum16{"PUMP2", "PUMP1"}."PUMP1", "HTS PORT IN"=w396) -> ("error out"=w398:errorcluster, "HTS PORT OUT"=w399:refnum<visa-resource-name>)  [unwired: 7 in]
                }
              }
            }
            n121 = Equal?(x=w369, y=0) -> (x = y?=w370:bool)
            n122 = case shown="False" w370 {
              tunnel: w378 -> [w411 _]
              tunnel: w369 -> [w410 _]
              tunnel: w376 -> [w404 w416]
              tunnel: [w403 w416] -> w375
              tunnel: w367 -> [w401 w415]
              tunnel: [w401 w415] -> w366
              frame False {
                n123 = Multiply(x=w410, y=6) -> (x*y=w402:i32)
                n124 = Number To Decimal String(number=w402) -> (decimal integer string=w408:string)  [unwired: 1 in]
                n125 = Concatenate Strings("PM1 OV3800A" ("Command"), w408, "EA0R" ("string")) -> (w405:string)
                n126 = call "HTS_WRITE_COMMAND.vi"("Error IN"=w404, "Command"=w405, "HTS PORT IN"=w411) -> ("Error OUT"=w413:errorcluster, "HTS PORT OUT"=w412:refnum<visa-resource-name>)  [unwired: 6 in, 1 out]
                n127 = call "wait_for_hts_pump.vi"("error in (no error)"=w413, "PUMP"=enum16{"PUMP2", "PUMP1"}."PUMP1", "HTS PORT IN"=w412) -> ("error out"=w403:errorcluster)  [unwired: 7 in, 1 out]
              }
              frame True {
              }
            }
          }
        }
      }
      n128 = call "move_and_wait.vi"("Error IN"=w325, "MOVE TO POSITION"=w322, "VISA Resource IN"=w323) -> ("Error OUT"=w324:errorcluster)  [unwired: 6 in, 2 out]
    }
    frame "INITIALIZE" {
      # "Move to valve to first reactor to sample"
      # "Empty syringe pump 2 into the cytometer, move to waste position\nprime the lines from pump1 to both media and stream selector"
      # "Move probe to sample \ninjection port"
      # "Initialize stream selector and\n the HTS probe motors and pumps"
      n129 = Get Notifier Status(notifier=w458, error in (no error)=w457) -> (notifier out=w455:refnum<notifier>, current notification=w456:T2, error out=w420:errorcluster)  [unwired: 2 out]
      n130 = Unbundle By Name(w456) -> ("REACTORS TO USE"=w423:u32[], "WASTE POSITION"=w444:i32, "HTS PORT"=w454:refnum<visa-resource-name>, "SELECTION VALVE PORT"=w417:refnum<visa-resource-name>)
      n131 = call "valve_init.vi"("error in (no error)"=w420, "VISA resource name"=w417) -> ("error out"=w453:errorcluster, "VISA resource name out"=w445:refnum<visa-resource-name>)  [unwired: 5 in, 2 out]
      n132 = call "HTS_WRITE_COMMAND.vi"("Error IN"=w453, "Command"="HOM", "HTS PORT IN"=w454) -> ("Error OUT"=w450:errorcluster, "HTS PORT OUT"=w451:refnum<visa-resource-name>)  [unwired: 6 in, 1 out]
      n133 = call "wait_for_hts_pump.vi"("error in (no error)"=w450, "PUMP"=enum16{"PUMP2", "PUMP1"}."PUMP1", "HTS PORT IN"=w451) -> ("error out"=w447:errorcluster, "HTS PORT OUT"=w446:refnum<visa-resource-name>)  [unwired: 7 in]
      n134 = call "wait_for_hts_pump.vi"("error in (no error)"=w447, "PUMP"=enum16{"PUMP2", "PUMP1"}."PUMP2", "HTS PORT IN"=w446) -> ("error out"=w438:errorcluster, "HTS PORT OUT"=w437:refnum<visa-resource-name>)  [unwired: 7 in]
      n135 = call "HTS_WRITE_COMMAND.vi"("Error IN"=w438, "Command"="GO Z 0", "HTS PORT IN"=w437) -> ("Error OUT"=w440:errorcluster, "HTS PORT OUT"=w441:refnum<visa-resource-name>)  [unwired: 6 in, 1 out]
      n136 = call "HTS_WAIT_FOR_READY.vi"("Error IN"=w440, "VISA resource IN"=w441) -> ("Error OUT"=w436:errorcluster, "VISA resource OUT"=w435:refnum<visa-resource-name>)  [unwired: 6 in, 2 out]
      n137 = call "HTS_WRITE_COMMAND.vi"("Error IN"=w436, "Command"="PM2 OA0IR", "HTS PORT IN"=w435) -> ("Error OUT"=w433:errorcluster, "HTS PORT OUT"=w434:refnum<visa-resource-name>)  [unwired: 6 in, 1 out]
      n138 = call "wait_for_hts_pump.vi"("error in (no error)"=w433, "PUMP"=enum16{"PUMP2", "PUMP1"}."PUMP2", "HTS PORT IN"=w434) -> ("error out"=w430:errorcluster, "HTS PORT OUT"=w426:refnum<visa-resource-name>)  [unwired: 7 in]
      n139 = call "move_and_wait.vi"("Error IN"=w430, "MOVE TO POSITION"=w444, "VISA Resource IN"=w445) -> ("Error OUT"=w443:errorcluster, "Visa Resource OUT"=w424:refnum<visa-resource-name>)  [unwired: 6 in, 1 out]
      n140 = call "HTS_WRITE_COMMAND.vi"("Error IN"=w443, "Command"="PM1 gOV5000A3000EA0G4R ", "HTS PORT IN"=w426) -> ("Error OUT"=w428:errorcluster, "HTS PORT OUT"=w429:refnum<visa-resource-name>)  [unwired: 6 in, 1 out]
      n141 = call "wait_for_hts_pump.vi"("error in (no error)"=w428, "PUMP"=enum16{"PUMP2", "PUMP1"}."PUMP1", "HTS PORT IN"=w429) -> ("error out"=w419:errorcluster)  [unwired: 7 in, 1 out]
      n142 = Index Array(array=w423, index=0) -> (element=w421:u32)
      n143 = call "move_and_wait.vi"("Error IN"=w419, "MOVE TO POSITION"=w421, "VISA Resource IN"=w424) -> ("Error OUT"=w418:errorcluster)  [unwired: 6 in, 2 out]
    }
    frame "CLEAR LINE TO CYTOMETER" {
      # "Pick up media with pump1\npush media/air bubble through\nthe line to pump2 -> cytometer"
      # "Set the valve \non PM2 \nto injection port\n-> cytometer"
      # "Move probe to injection port"
      n144 = Get Notifier Status(notifier=w467, error in (no error)=w466) -> (notifier out=w464:refnum<notifier>, current notification=w465:T2, error out=w459:errorcluster)  [unwired: 2 out]
      n145 = Unbundle By Name(w465) -> ("HTS PORT"=w463:refnum<visa-resource-name>)
      n146 = call "HTS_WRITE_COMMAND.vi"("Error IN"=w459, "Command"="GO Z 0", "HTS PORT IN"=w463) -> ("Error OUT"=w482:errorcluster, "HTS PORT OUT"=w483:refnum<visa-resource-name>)  [unwired: 6 in, 1 out]
      n147 = call "HTS_WAIT_FOR_READY.vi"("Error IN"=w482, "VISA resource IN"=w483) -> ("Error OUT"=w481:errorcluster, "VISA resource OUT"=w480:refnum<visa-resource-name>)  [unwired: 6 in, 2 out]
      n148 = call "load_bubble.vi"("error in (no error)"=w481, "HTS PORT"=w480) -> ("error out"=w470:errorcluster, "HTS PORT OUT"=w471:refnum<visa-resource-name>)  [unwired: 8 in]
      n149 = call "HTS_WRITE_COMMAND.vi"("Error IN"=w470, "Command"="PM2 BR", "HTS PORT IN"=w471) -> ("Error OUT"=w473:errorcluster, "HTS PORT OUT"=w474:refnum<visa-resource-name>)  [unwired: 6 in, 1 out]
      n150 = call "wait_for_hts_pump.vi"("error in (no error)"=w473, "PUMP"=enum16{"PUMP2", "PUMP1"}."PUMP2", "HTS PORT IN"=w474) -> ("error out"=w462:errorcluster, "HTS PORT OUT"=w468:refnum<visa-resource-name>)  [unwired: 7 in]
      n151 = call "HTS_WRITE_COMMAND.vi"("Error IN"=w462, "Command"="PM1 V2400OA3000EA0R", "HTS PORT IN"=w468) -> ("Error OUT"=w477:errorcluster, "HTS PORT OUT"=w476:refnum<visa-resource-name>)  [unwired: 6 in, 1 out]
      n152 = call "wait_for_hts_pump.vi"("error in (no error)"=w477, "PUMP"=enum16{"PUMP2", "PUMP1"}."PUMP1", "HTS PORT IN"=w476) -> ("error out"=w461:errorcluster)  [unwired: 7 in, 1 out]
    }
  }
  "error out" <- w6
  "Settings" <- w5
  "EXP Settings" <- w4
